vi "Populate Available Objects for PDO Mapping.vi"(8 "error in":errorcluster, 10 "Type":enum16{"TX PDO", "RX PDO"}(ring), 11 "UI Actor in":refnum<class "UI Actor.lvclass">) -> (0 "error out":errorcluster, 3 "UI Actor out":refnum<class "UI Actor.lvclass">)   [LabVIEW 2024, in "UI Actor.lvlib" / "UI Actor.lvclass"]
uses:
  UI Actor.lvclass
  UI Actor.lvclass/UI Actor.ctl
  Core/OD Sub-Entry/OD Sub-Entry.lvclass
  D:/git/EDS-File-Viewer/source/Core/OD Entry/OD Entry.lvclass
  Electronic Datasheet/Electronic Datasheet.lvclass
  Core/OD Entry/OD Entry.lvclass
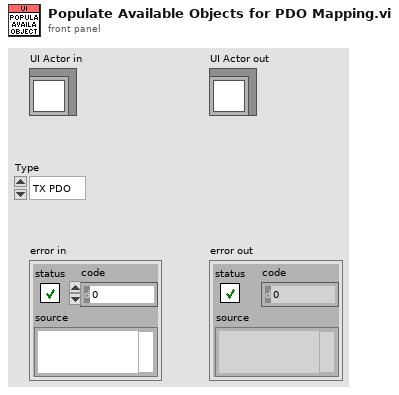
[diagram p1: front panel]
types:
  T1 = map{path, refnum<class "Electronic Datasheet.lvclass">}
  T2 = enum16{"UNKNOWN", "BOOLEAN", "INTEGER8", "INTEGER16", "INTEGER32", "UNSIGNED8", "UNSIGNED16", "UNSIGNED32", "REAL32", "VISIBLE_STRING", "OCTET_STRING", "UNICODE_STRING", "TIME_OF_DAY", "TIME_DIFFERENCE", "RESERVED1", "DOMAIN", "INTEGER24", "REAL64", "INTEGER40", "INTEGER48", "INTEGER56", "INTEGER64", "UNSIGNED24", "RESERVED2", "UNSIGNED40", "UNSIGNED48", "UNSIGNED56", "UNSIGNED64", "RESERVED3", "RESERVED4", "RESERVED5", "RESERVED6", "PDO_COMMUNICATION_PARAMETER", "PDO_MAPPING", "SDO_PARAMETER", "IDENTITY", "RESERVED7"}
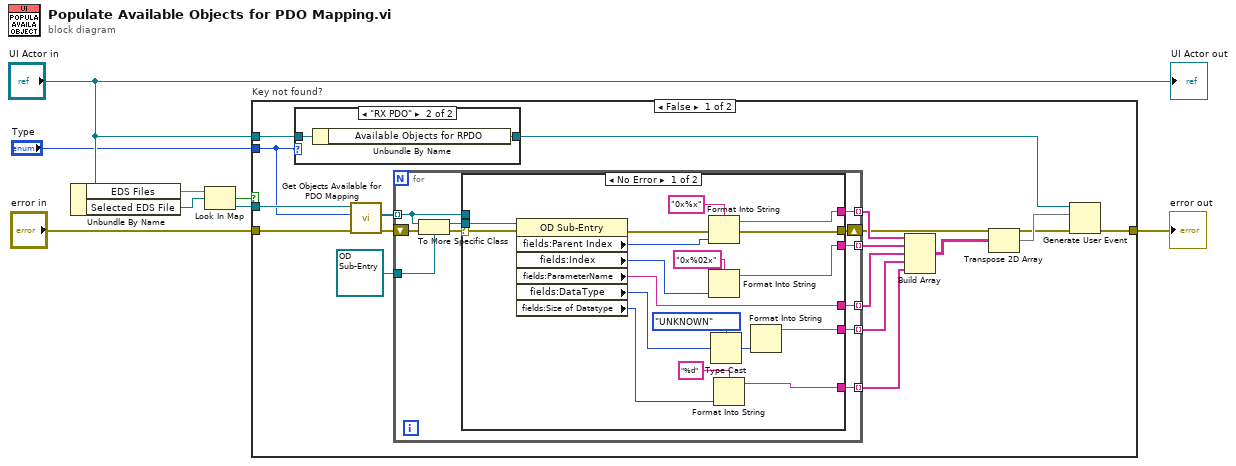
[diagram p0: block diagram]
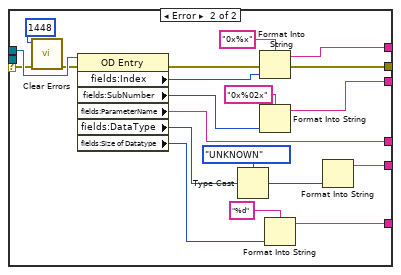
[diagram p2: hidden frame]
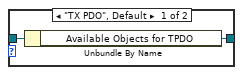
[diagram p3: hidden frame]
diagram:
  n1 = Unbundle By Name("UI Actor in") -> ("EDS Files"=w8:T1, "Selected EDS File"=w7:path)
  n2 = Look In Map(map=w8, key=w7) -> (key not found?=w6:bool, value=w5:refnum<class "Electronic Datasheet.lvclass">)  [unwired: 1 in]
  n3 = case "Key not found?" shown="False" w6 {
    tunnel: w5 -> [w25 _]
    tunnel: "error in" -> [w24 w79]
    tunnel: [w16 w79] -> w2
    tunnel: "UI Actor in" -> [w12 _]
    tunnel: "Type" -> [w11 _]
    frame False {
      n4 = case shown="\"RX PDO\"" w11 {
        tunnel: [w75 w78] -> w21
        tunnel: w12 -> [w76 w77]
        frame "TX PDO", Default {
          n5 = Unbundle By Name(w76) -> ("Available Objects for TPDO"=w75:refnum<user-event>)
        }
        frame "RX PDO" {
          n6 = Unbundle By Name(w77) -> ("Available Objects for RPDO"=w78:refnum<user-event>)
        }
      }
      n7 = call "Get Objects Available for PDO Mapping.vi"("Error In"=w24, "Type"=w11, "reference in"=w25) -> ("Error Out"=w22:errorcluster, "Objects Available for PDO Mapping"=w23:refnum<class "OD Entry.lvclass">[])  [unwired: 6 in, 1 out]
      n8 = for {
        tunnel: w23 -> [w30] mode=indexing
        tunnel: [w35] -> w18 mode=indexing
        shift-right: [w34] -> w17
        shift-left: w22 -> [w29]
        tunnel: [w36] -> w19 mode=indexing
        tunnel: [w33] -> w15 mode=indexing
        tunnel: [w32] -> w14 mode=indexing
        tunnel: [w31] -> w13 mode=indexing
        tunnel: refnum<class "OD Sub-Entry.lvclass"> refnum ("Electronic Datasheet.lvlib:OD Sub-Entry") -> [w27]
        n9 = To More Specific Class(target class=w27, reference=w30, error in=w29) -> (specific class reference=w26:refnum<class "OD Sub-Entry.lvclass">, error out=w28:errorcluster)
        n10 = case shown="No Error" w28 {
          selector: w28 -> [w45 w61]
          tunnel: [w41 w73] -> w36
          tunnel: [w40 w69] -> w35
          tunnel: [w44 w67] -> w34
          tunnel: [w42 w66] -> w33
          tunnel: [w39 w65] -> w32
          tunnel: [w38 w63] -> w31
          tunnel: w30 -> [_ w62]
          tunnel: w26 -> [w43 _]
          frame No Error {
            n11 = property class="OD Sub-Entry"(reference=w43, error in=w45) -> (error out=w50:errorcluster, "fields:Parent Index"=w53:u16, "fields:Index"=w51:u16, "fields:ParameterName"=w42:string, "fields:DataType"=w49:u16, "fields:Size of Datatype"=w48:i32)  [unwired: 1 out]
            n12 = Format Into String(format string="0x%x", error in=w50, w53) -> (resulting string=w41:string, error out=w44:errorcluster)  [unwired: 1 in]
            n13 = Format Into String(format string="0x%02x", w51) -> (resulting string=w40:string)  [unwired: 2 in, 1 out]
            n14 = Type Cast(type=T2."UNKNOWN" ("DataType"), x=w49) -> (*(type *) &x=w46:T2)
            n15 = Format Into String(format string="%d", w48) -> (resulting string=w38:string)  [unwired: 2 in, 1 out]
            n16 = Format Into String(w46) -> (resulting string=w39:string)  [unwired: 3 in, 1 out]
          }
          frame Error {
            n17 = call <vilib>:"Clear Errors.vi"("error in (no error)"=w61, "specific error code to clear (0: all)"=1448) -> ("error out"=w60:errorcluster)  [unwired: 4 in, 1 out]
            n18 = property class="OD Entry"(reference=w62, error in=w60) -> (error out=w68:errorcluster, "fields:Index"=w72:u16, "fields:SubNumber"=w70:u8, "fields:ParameterName"=w66:string, "fields:DataType"=w57:u16, "fields:Size of Datatype"=w64:i32)  [unwired: 1 out]
            n19 = Type Cast(type=T2."UNKNOWN" ("DataType"), x=w57) -> (*(type *) &x=w56:T2)
            n20 = Format Into String(format string="0x%x", error in=w68, w72) -> (resulting string=w73:string, error out=w67:errorcluster)  [unwired: 1 in]
            n21 = Format Into String(format string="0x%02x", w70) -> (resulting string=w69:string)  [unwired: 2 in, 1 out]
            n22 = Format Into String(format string="%d", w64) -> (resulting string=w63:string)  [unwired: 2 in, 1 out]
            n23 = Format Into String(w56) -> (resulting string=w65:string)  [unwired: 3 in, 1 out]
          }
        }
      }
      n24 = Build Array(w19, w18, w15, w14, w13) -> (w10:string[][])
      n25 = Transpose 2D Array(2D array=w10) -> (transposed array=w20:string[][])
      n26 = Generate User Event(user event=w21, event data cluster=w20, error in=w17) -> (error out=w16:errorcluster)  [unwired: 1 in, 1 out]
    }
    frame True {
    }
  }
  "error out" <- w2
  "UI Actor out" <- "UI Actor in"
